vi "Get Config.vi"(6 "?":T1=enum."path", 8 "error in (no error)":errorcluster, 9 "section":string, 10 "key":string, 11 "Config in":refnum<class "Config.lvclass">) -> (0 "error out":errorcluster, 1 "found?":bool, 2 "Data":variant, 3 "Config out":refnum<class "Config.lvclass">)   [LabVIEW 2018, in "Config.lvlib" / "Config.lvclass"]
uses:
  Config.lvclass
  Controls/KeyType.ctl
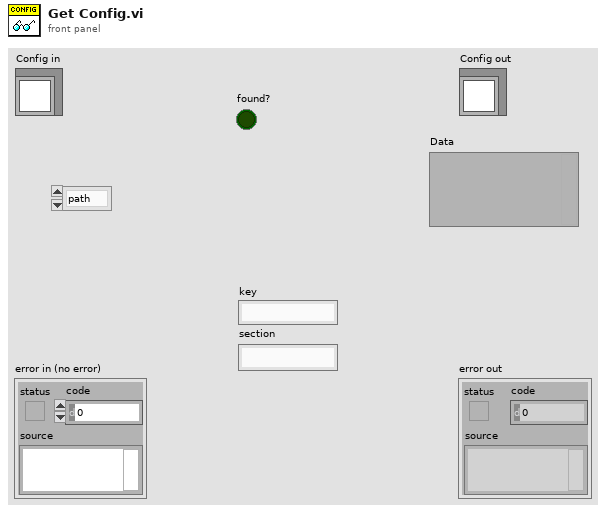
[diagram p1: front panel]
types:
  T1 = typedef "Config.lvlib/Config.lvclass/KeyType.ctl" = enum16{"dbl", "path", "string ", "u32", "i32", "boolean"}
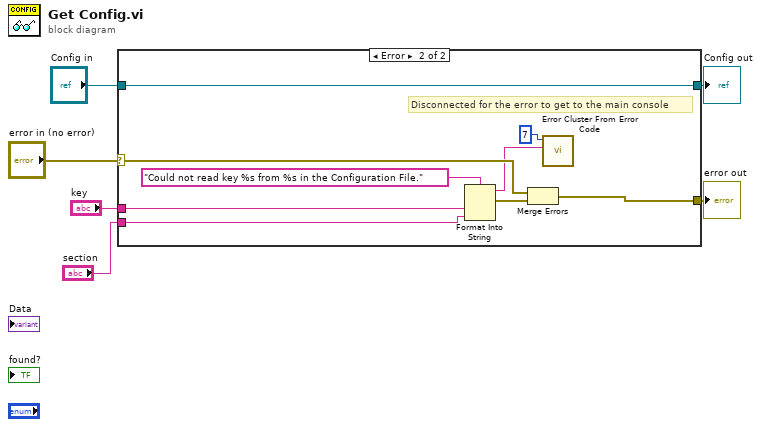
[diagram p0: block diagram]
diagram:
  n1 = case shown="Error" "error in (no error)" {
    selector: "error in (no error)" -> [w7 w15]
    tunnel: [w7 w10] -> w5
    tunnel: [w8 w17] -> w3
    tunnel: "Config in" -> [w8 w17]
    tunnel: "key" -> [_ w13]
    tunnel: "section" -> [_ w12]
    frame No Error {
      # "Abstract method.\nNO CODE HERE."
      # "Wire the error cluster across even in the \"No Error\"\ncase so that warnings get propagated."
    }
    frame Error {
      # "Disconnected for the error to get to the main console"
      n2 = Format Into String(format string="Could not read key %s from %s in the Configuration File." ("error message (\"\")"), w13, w12) -> (resulting string=w14:string, error out=w9:errorcluster)  [unwired: 2 in]
      n3 = Merge Errors(w15, w9) -> (w10:errorcluster)
      n4 = call <vilib>:"Error Cluster From Error Code.vi"("error message (\"\")"=w14, "error code (0)"=7) -> ()  [unwired: 7 in, 1 out]
    }
  }
  "error out" <- w5
  "Config out" <- w3
